vi "Disconnect.vi"(7 "error in (no error)":errorcluster, 10 "Motion in":refnum<class "Motion.lvclass">) -> (0 "error out":errorcluster)   [LabVIEW 2016, in "Motion.lvclass"]
uses:
  Motion.lvclass
  Controller Folder/Controller.lvclass
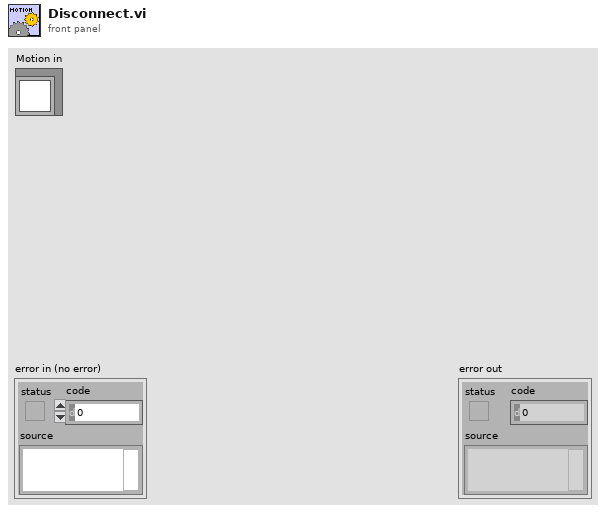
[diagram p1: front panel]
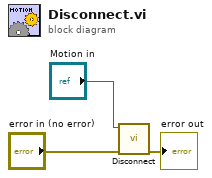
[diagram p0: block diagram]
diagram:
  n1 = call-parent "Disconnect.vi"("error in (no error)"="error in (no error)", "Controller in"="Motion in") -> ("error out"=→"error out":errorcluster)  [unwired: 8 in]
